vi "AskNodeForServiceProviders.vi"(0 "Service ROS":T5={"topic port"=0, "Node"="", "topic"="", "type"="", "node port"=0, "error "={"status"=FALSE, "code"=0, "source"=""}, "Direction"=enum."Node", "APIs"=[], "Update (ms)"=1, "write queue"=1}) -> (1 "Connections":T2(array[cluster]), 2 "MyState":T4, 3 "Log":T1, 4 "error out":errorcluster)   [LabVIEW 2012]
uses:
  _ROSDefinition.vi
  SubVIs/_ROSDirection.ctl
  SubVIs/_ROSControl.ctl
  MyState.ctl
  ROSLog.ctl
panel:
  out "Reply":T3(array[cluster])
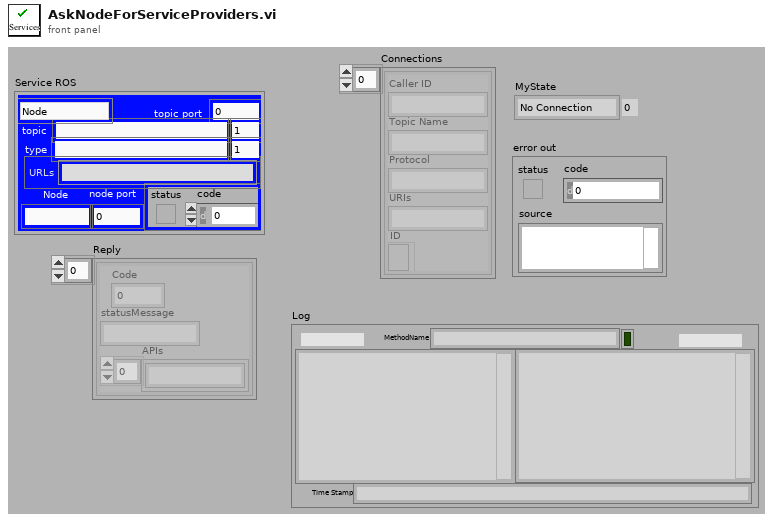
[diagram p1: front panel]
types:
  T1 = typedef "ROSLog.ctl" = cluster{"Sent":string, "Reply":string, "MethodName":string, "success":bool, "Dir1":string, "Dir2":string, "Time Stamp":string}
  T2 = cluster{"Caller ID":string, "Topic Name":string, "Protocol":string, "URIs":string, "ID":refnum<k5>}[]
  T3 = cluster{"Code":i8, "statusMessage":string, "APIs":string[]}[]
  T4 = typedef "MyState.ctl" = enum16{"No Connection", "Registered", "Connected", "Close"}
  T5 = typedef "_ROSControl.ctl" = cluster{"topic port":u16, "Node":string, "topic":string, "type":string, "node port":u32, "error ":errorcluster, "Direction":T6, "APIs":string[], "Update (ms)":u16, "write queue":u16}
  T6 = typedef "_ROSDirection.ctl" = enum16{"Node", "Publisher", "Subscriber", "Service Client"}
  T7 = cluster{"Caller ID":string, "Topic Name":string, "Protocol":string, "URIs":string, "ID":refnum<k5>}
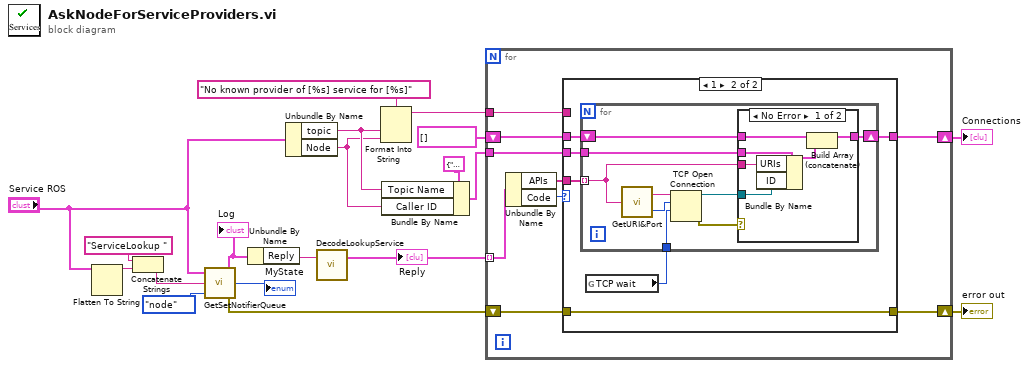
[diagram p0: block diagram]
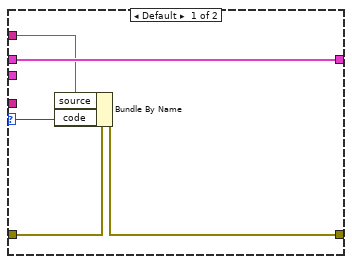
[diagram p2: hidden frame]
diagram:
  n1 = Flatten To String(anything="Service ROS") -> (data string=w17:string)  [unwired: 3 in, 2 out]
  n2 = Concatenate Strings("ServiceLookup " ("element"), w17) -> (w16:string)
  n3 = call "GetSetNotifierQueue.vi"("Name"=enum16{"topic", "node"}."node", "Command"=w16, "ROS"="Service ROS") -> ("error out"=w1:errorcluster, "MyState"=→"MyState":T4, "Log"=w14:T1)
  "Log" <- w14
  n4 = Unbundle By Name(w14) -> ("Reply"=w13:string)
  n5 = Unbundle By Name("Service ROS") -> ("topic"=w10:string, "Node"=w9:string)
  n6 = call "DecodeLookupService.vi"("Response"=w13) -> ("Reply"=w5:T3)  [unwired: 1 in, 1 out]
  "Reply" <- w5
  n7 = Format Into String(format string="No known provider of [%s] service for [%s]", w10, w9) -> (resulting string=w6:string)  [unwired: 2 in, 1 out]
  n8 = Bundle By Name(cluster=T7 {"Caller ID"="", "Topic Name"="", "Protocol"="???", "URIs"="", "ID"=refnum} ("Subscriber"), "Topic Name"=w10, "Caller ID"=w9) -> (w8:T7)
  n9 = for {
    tunnel: w5 -> [w28] mode=indexing
    shift-right: [w21] -> w3
    shift-left: w1 -> [w20]
    tunnel: w8 -> [w26]
    shift-right: [w24] -> w4
    shift-left: T2 [] -> [w25]
    tunnel: w6 -> [w22]
    n10 = Unbundle By Name(w28) -> ("APIs"=w27:string[], "Code"=w23:i8)
    n11 = case shown="1" w23 {
      selector: w23 -> [w31 _]
      tunnel: w27 -> [_ w39]
      tunnel: w26 -> [_ w38]
      tunnel: w25 -> [w33 w37]
      tunnel: [w33 w36] -> w24
      tunnel: w22 -> [w32 _]
      tunnel: [w29 w35] -> w21
      tunnel: w20 -> [w30 w35]
      frame Default {
        n12 = Bundle By Name(cluster=w30, "source"=w32, "code"=w31) -> (w29:errorcluster)
      }
      frame 1 {
        n13 = global read "_ROSDefinition.vi" "TCP wait"() -> (w34:i32)
        n14 = for {
          tunnel: w39 -> [w41] mode=indexing
          tunnel: w38 -> [w42]
          shift-right: [w45] -> w36
          shift-left: w37 -> [w44]
          tunnel: w34 -> [w40]
          n15 = call "GetURI&Port.vi"("URI in"=w41) -> ("Port"=w48:u16, "URI"=w47:string)
          n16 = TCP Open Connection(address=w47, remote port or service name=w48, timeout ms (60000)=w40) -> (connection ID=w43:refnum<k5>, error out=w46:errorcluster)  [unwired: 2 in]
          n17 = case shown="No Error" w46 {
            tunnel: [w54 w55] -> w45
            tunnel: w44 -> [w53 w55]
            tunnel: w43 -> [w50 _]
            tunnel: w42 -> [w52 _]
            tunnel: w41 -> [w51 _]
            frame No Error {
              n18 = Bundle By Name(cluster=w52, "URIs"=w51, "ID"=w50) -> (w49:T7)
              n19 = Build Array (concatenate)(w53, w49) -> (w54:T2)
            }
            frame Error {
            }
          }
        }
      }
    }
  }
  "Connections" <- w4
  "error out" <- w3
